vi "Periodic Tasks.vi"(9 "error out 3":errorcluster) -> ()   [LabVIEW 2012]
doc: "This VI runs in parallel to other tasks. It can contain as many user-defined periodic loops as you need. These can carry out PID or other sorts of timed response."
uses:
  <vilib>/Rock Robotics/WPI/DriverStation/DriverStationLCD/WPI_DriverStationLCDLCDLine.ctl
panel:
  in  "pidGains":T1={"proportional gain (Kc)"=1.0, "integral time (Ti, min)"=0.01, "derivative time (Td, min)"=0.0} {"derivative time (Td, min)" format="%.3f"; "integral time (Ti, min)" format="%.3f"; "proportional gain (Kc)" format="%.3f"}
  in  "Requested RPM":dbl
  in  "Method Selection2":enum16{"Manual", "PID", "BangBang"}(ring)
  in  "Multiplier":dbl
  in  "milliseconds to wait":u32
  out "Average Difference":dbl
  out "RPM":dbl
  out "Period (sec)":dbl
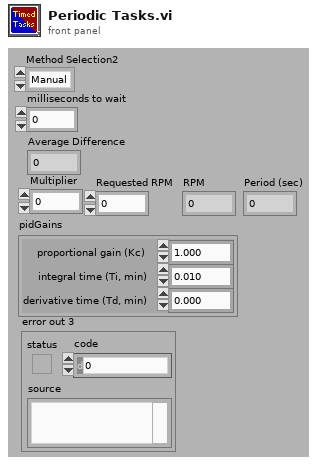
[diagram p1: front panel]
types:
  T1 = cluster{"proportional gain (Kc)":dbl, "integral time (Ti, min)":dbl, "derivative time (Td, min)":dbl}
  T2 = typedef "WPI_CounterDevRef.ctl" = cluster{"DevStatus":errorcluster, "CntIndex":T3}
  T3 = typedef "FPGA_CounterCtrSystemIndex.ctl" = enum8{"Ctr 0", "Ctr 1", "Ctr 2", "Ctr 3", "Ctr 4", "Ctr 5", "Ctr 6", "Ctr 7", "Invalid"}
  T4 = typedef "WPI_MotorControlDeviceRef.ctl" = cluster{"DeviceStatus":errorcluster, "Type":enum16{"PWM", "CAN"}, "PWM":cluster{"Digital Module":T5, "PWM Channel":T6, "DeadBand":T7}, "CAN":cluster{"Device Number":u8, "Control Mode":T8, "Semaphore":T9, "Max Vout":dbl}, "Invert":bool, "TransformRef":T10, "InvTransformRef":T10}
  T5 = typedef "FPGA_TypedefDigitalModule.ctl" = enum16{"Digital Module 1", "Digital Module 2"}
  T6 = typedef "FPGA_DIOPWMChannel.ctl" = enum8{"PWM 1", "PWM 2", "PWM 3", "PWM 4", "PWM 5", "PWM 6", "PWM 7", "PWM 8", "PWM 9", "PWM 10", "Invalid"}
  T7 = typedef "WPI_PWMDeadband.ctl" = cluster{"Name":string, "maxPositivePwm":i32, "minPositivePwm":i32, "centerPwm":i32, "maxNegativePwm":i32, "minNegativePwm":i32, "angularRange":u16}
  T8 = typedef "WPI_CANJaguar_ControlMode.ctl" = enum8{"Percent VBus", "Current", "Speed", "Position", "Voltage"}
  T9 = typedef "Semaphore RefNum" = refnum<k1>
  T10 = typedef "WPI_PWMTransform_ConPane.ctl" = refnum<vi>
  T11 = typedef "WPI_DriverStationLCDLCDLine.ctl" = enum16{"Main - Line 1", "User - Line 2", "User - Line 3", "User - Line 4", "User - Line 5", "User - Line 6"}
  T12 = cluster{"[0]":dbl, "[1]":dbl, "[2]":dbl, "[3]":dbl, "[4]":dbl, "[5]":dbl, "[6]":dbl, "[7]":dbl, "[8]":dbl}
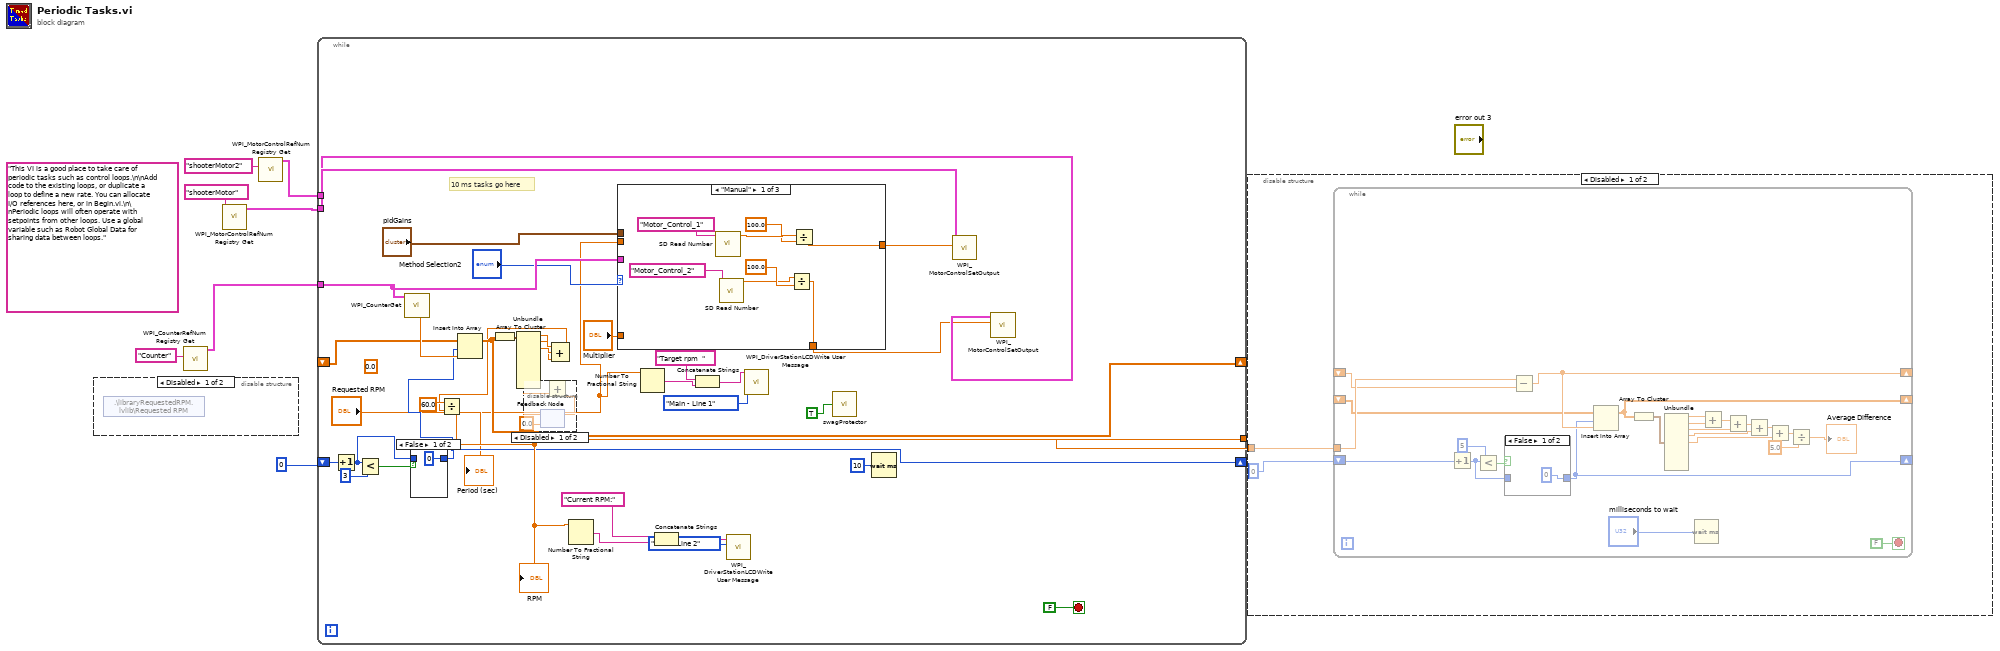
[diagram p0: block diagram]
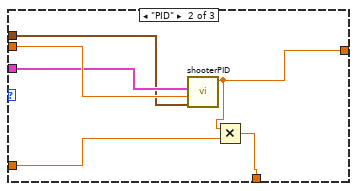
[diagram p7: hidden frame]
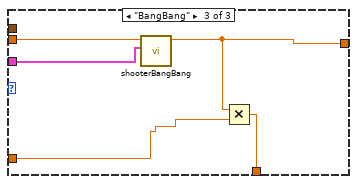
[diagram p8: hidden frame]
diagram:
  (unwired) "This VI is a good place to take care of periodic tasks such as control loops.\n\nAdd code to the existing loops, or duplicate a loop to define a new rate. You can allocate I/O references here, or in Begin.vi.\n\nPeriodic loops will often operate with setpoints from other loops. Use a global variable such as Robot Global Data for sharing data between loops."
  n1 = disable-structure shown="Disabled" {
    frame Disabled {
      n2 = shared-variable ".\\libraryRequestedRPM.lvlib\\Requested RPM"() -> (w9:dbl)  [unwired: 1 in, 1 out]
    }
    frame Enabled {
    }
  }
  n3 = call <vilib>:"WPI_CounterRefNum Registry Get.vi"("refnum name"="Counter") -> ("CounterDevRef"=w8:T2)  [unwired: 9 in, 1 out]
  n4 = call <vilib>:"WPI_MotorControlRefNum Registry Get.vi"("refnum name"="shooterMotor") -> ("MotorControlDevRef"=w7:T4)  [unwired: 9 in, 1 out]
  n5 = call <vilib>:"WPI_MotorControlRefNum Registry Get.vi"("refnum name"="shooterMotor2") -> ("MotorControlDevRef"=w3:T4)  [unwired: 9 in, 1 out]
  n6 = while {
    tunnel: w8 -> [w26]
    tunnel: w7 -> [w42]
    tunnel: [w34] -> w2
    tunnel: w3 -> [w36]
    shift-right: [w23] -> _
    shift-left: _ -> [w22]
    shift-right: [w17] -> _
    shift-left: 0 -> [w21]
    stop <- FALSE stop-if-true
    (unwired) 0.0 ("x")
    # "10 ms tasks go here"
    n7 = Increment(x=w21) -> (x+1=w18:i32)
    n8 = Less?(x=w18, y=3) -> (x < y?=w19:bool)
    n9 = call <vilib>:"WPI_CounterGet.vi"("CounterDevRef in"=w26) -> ("Period (sec)"=w24:dbl)  [unwired: 5 in, 5 out]
    n10 = case shown="False" w19 {
      tunnel: w18 -> [_ w49]
      tunnel: [0 w49] -> w17
      frame False {
      }
      frame True {
      }
    }
    n11 = Insert Into Array(array=w22, index=w17, new element=w24) -> (w23:dbl[])
    n12 = Array To Cluster(array=w23) -> (cluster=w16:T12)
    n13 = Unbundle(w16) -> ("[0]"=w15:dbl, "[1]"=w14:dbl, "[2]"=w13:dbl)  [unwired: 6 out]
    n14 = disable-structure shown="Disabled" {
      frame Disabled {
        n15 = feedback #1(0.0) -> (w47:dbl)
        n16 = Add(y=w47) -> (x+y=w45:dbl)  [unwired: 1 in]
        n17 = feedback-in #1(w45) -> ()
      }
      frame Enabled {
      }
    }
    n18 = Compound Arithmetic op=ADD(w15, w14, w13) -> (w12:dbl)
    "Period (sec)" <- w12
    n19 = Divide(x=60.0, y=w12) -> (x/y=w34:dbl)
    "RPM" <- w34
    n20 = Number To Fractional String(number=w34) -> (F-format string=w35:string)  [unwired: 3 in]
    n21 = case shown="\"Manual\"" "Method Selection2" {
      tunnel: [w55 w61 w68] -> w29
      tunnel: [w54 w59 w67] -> w28
      tunnel: "Multiplier" -> [_ w60 w66]
      tunnel: w26 -> [_ w62 w65]
      tunnel: "Requested RPM" -> [_ w63 w64]
      tunnel: "pidGains" -> [_ w58 _]
      frame "Manual" {
        n22 = call <vilib>:"SD Read Number.vi"("Name"="Motor_Control_1") -> ("Numeric"=w51:dbl)  [unwired: 8 in, 2 out]
        n23 = call <vilib>:"SD Read Number.vi"("Name"="Motor_Control_2") -> ("Numeric"=w52:dbl)  [unwired: 8 in, 2 out]
        n24 = Divide(x=w52, y=100.0) -> (x/y=w54:dbl)
        n25 = Divide(x=w51, y=100.0) -> (x/y=w55:dbl)
      }
      frame "PID" {
        n26 = call "shooterPID.vi"("pidGains"=w58, "rpmTarget"=w63, "CounterDevRef"=w62) -> ("output"=w61:dbl)  [unwired: 8 in]
        n27 = Multiply(x=w61, y=w60) -> (x*y=w59:dbl)
      }
      frame "BangBang" {
        n28 = call "shooterBangBang.vi"("CounterDevRef in"=w65, "rpmTarget"=w64) -> ("Output"=w68:dbl)  [unwired: 9 in]
        n29 = Multiply(x=w68, y=w66) -> (x*y=w67:dbl)
      }
    }
    n30 = Number To Fractional String(number="Requested RPM") -> (F-format string=w41:string)  [unwired: 3 in]
    n31 = Concatenate Strings("Current RPM:" ("string"), w35) -> (w33:string)
    n32 = Concatenate Strings("Target rpm  " ("string"), w41) -> (w39:string)
    n33 = call <vilib>:"WPI_DriverStationLCDWrite User Message.vi"("line text"=w33, "line"=WPI_DriverStationLCDLCDLine."User - Line 2") -> ()  [unwired: 13 in, 1 out]
    n34 = call <vilib>:"WPI_DriverStationLCDWrite User Message.vi"("line text"=w39, "line"=WPI_DriverStationLCDLCDLine."Main - Line 1") -> ()  [unwired: 13 in, 1 out]
    n35 = call "swagProtector.vi"("enabled?"=TRUE) -> ()  [unwired: 2 in]
    n36 = Wait (ms)(milliseconds to wait=u32 10) -> ()  [unwired: 1 out]
    n37 = call <vilib>:"WPI_MotorControlSetOutput.vi"("Output"=w29, "MotorControlDevRef"=w42) -> ()  [unwired: 7 in, 3 out]
    n38 = call <vilib>:"WPI_MotorControlSetOutput.vi"("Output"=w28, "MotorControlDevRef"=w36) -> ()  [unwired: 7 in, 3 out]
  }
  n39 = disable-structure shown="Disabled" {
    disable-tunnel: w2 -> [w69 _]
    frame Disabled {
      n40 = while {
        tunnel: w69 -> [w94]
        shift-right: [w92] -> _
        shift-left: _ -> [w93]
        shift-right: [w87] -> _
        shift-left: _ -> [w91]
        shift-right: [w79] -> _
        shift-left: 0 -> [w78]
        stop <- FALSE stop-if-true
        n41 = Increment(x=w78) -> (x+1=w88:i32)
        n42 = Less?(x=w88, y=5) -> (x < y?=w89:bool)
        n43 = case shown="False" w89 {
          tunnel: w88 -> [_ w96]
          tunnel: [0 w96] -> w79
          frame False {
          }
          frame True {
          }
        }
        n44 = Subtract(x=w94, y=w93) -> (x-y=w92:dbl)
        n45 = Insert Into Array(array=w91, index=w79, new element=w92) -> (w87:dbl[])
        n46 = Array To Cluster(array=w87) -> (cluster=w86:T12)
        n47 = Unbundle(w86) -> ("[0]"=w84:dbl, "[1]"=w85:dbl, "[2]"=w82:dbl, "[3]"=w80:dbl, "[4]"=w76:dbl)  [unwired: 4 out]
        n48 = Wait (ms)(milliseconds to wait="milliseconds to wait") -> ()  [unwired: 1 out]
        n49 = Add(x=w84, y=w85) -> (x+y=w83:dbl)
        n50 = Add(x=w83, y=w82) -> (x+y=w81:dbl)
        n51 = Add(x=w81, y=w80) -> (x+y=w77:dbl)
        n52 = Add(x=w77, y=w76) -> (x+y=w75:dbl)
        n53 = Divide(x=w75, y=5.0) -> (x/y=→"Average Difference":dbl)
      }
    }
    frame Enabled {
    }
  }
